vi "ArduinoParse.vi"(0 "read buffer":string, 1 "Expected Arduino Parameters":i32=8) -> (2 "Number Arduino Parameters":i32, 3 "Arduino Data Names":string[](array[string]), 4 "Arduino Data":dbl[](array[numeric]), 5 "Arduino Read Failed?":bool)   [LabVIEW 2012]
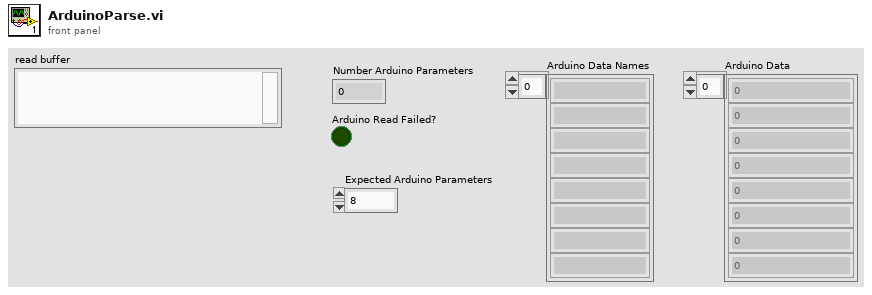
[diagram p1: front panel]
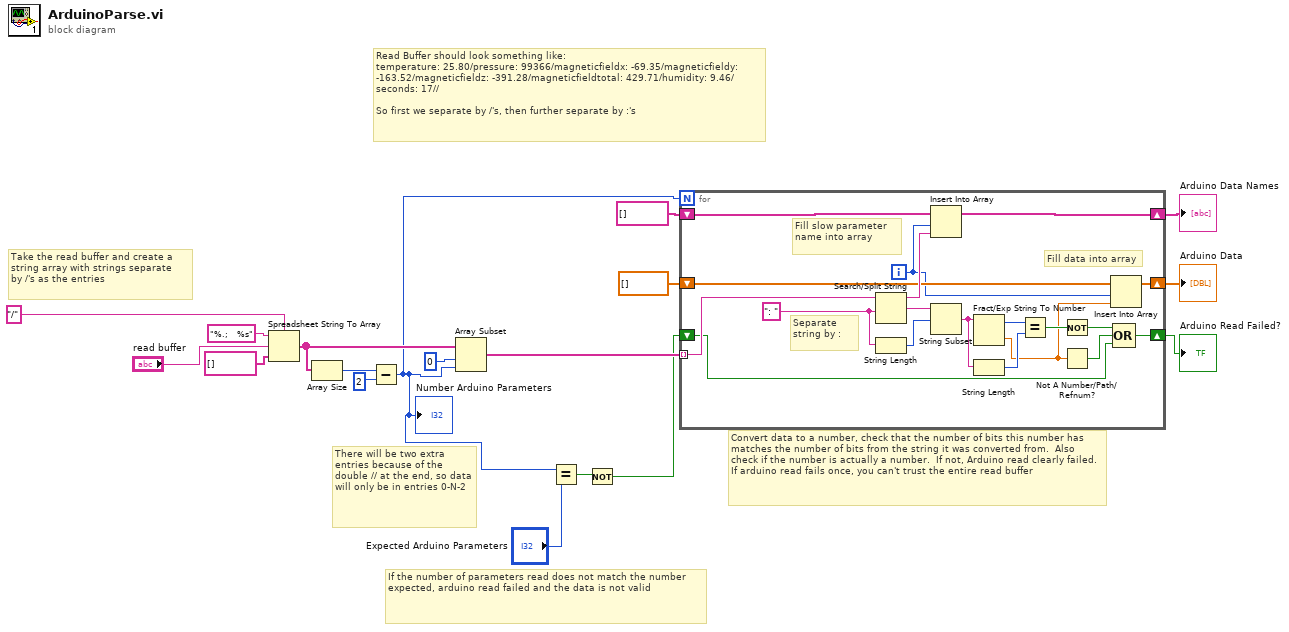
[diagram p0: block diagram]
diagram:
  # "If the number of parameters read does not match the number expected, arduino read failed and the data is not valid"
  # "Convert data to a number, check that the number of bits this number has matches the number of bits from the string it was converted from.  Also check if the number is actually a number.  If not, Arduino read clearly failed.  If arduino read fails once, you can't trust the entire read buffer"
  # "Read Buffer should look something like:\ntemperature: 25.80/pressure: 99366/magneticfieldx: -69.35/magneticfieldy: -163.52/magneticfieldz: -391.28/magneticfieldtotal: 429.71/humidity: 9.46/seconds: 17//\n\nSo first we separate by /'s, then further separate by :'s"
  # "There will be two extra entries because of the double // at the end, so data will only be in entries 0-N-2"
  # "Take the read buffer and create a string array with strings separate by /'s as the entries"
  n1 = Spreadsheet String To Array(delimiter (Tab)="/", format string="%.;   %s", spreadsheet string="read buffer", array type (2D Dbl)=string[] []) -> (array=w13:string[])
  n2 = Array Size(array=w13) -> (size(s)=w12:i32)
  n3 = Subtract(x=w12, y=2) -> (x-y=w4:i32)
  "Number Arduino Parameters" <- w4
  n4 = Array Subset(array=w13, index=0, length=w4) -> (w8:string[])
  n5 = Equal?(x=w4, y="Expected Arduino Parameters") -> (x = y?=w2:bool)
  n6 = Not(x=w2) -> (.not. x?=w1:bool)
  n7 = for {
    N: w4 -> [_]
    shift-right: [w29] -> w7
    shift-left: string[] [] ("array type (2D Dbl)") -> [w31]
    shift-right: [w21] -> w5
    shift-left: dbl[] [] ("array type (2D Dbl)") -> [w24]
    tunnel: w8 -> [w32] mode=indexing
    shift-right: [w26] -> w6
    shift-left: w1 -> [w25]
    i -> [w23]
    w20 = ": " ("search string/char (-)")
    # "Fill data into array"
    # "Fill slow parameter name into array"
    # "Separate string by :"
    n8 = Search/Split String(string=w32, search string/char (-)=w20) -> (substring before match=w30:string, match + rest of string=w33:string)  [unwired: 1 in, 1 out]
    n9 = String Length(string=w20) -> (length=w19:i32)
    n10 = Insert Into Array(array=w31, index=w23, new element=w30) -> (w29:string[])
    n11 = String Subset(string=w33, offset (0)=w19) -> (substring=w34:string)  [unwired: 1 in]
    n12 = Fract/Exp String To Number(string=w34) -> (offset past number=w37:i32, number=w22:dbl)  [unwired: 3 in]
    n13 = String Length(string=w34) -> (length=w36:i32)
    n14 = Equal?(x=w37, y=w36) -> (x = y?=w35:bool)
    n15 = Not(x=w35) -> (.not. x?=w28:bool)
    n16 = Not A Number/Path/Refnum?(number/path/refnum=w22) -> (NaN/Path/Refnum?=w27:bool)
    n17 = Insert Into Array(array=w24, index=w23, new element=w22) -> (w21:dbl[])
    n18 = Compound Arithmetic op=OR(w28, w27, w25) -> (w26:bool)
  }
  "Arduino Data Names" <- w7
  "Arduino Read Failed?" <- w6
  "Arduino Data" <- w5
